vi "EPS-Remote Mode.vi"(8 "error in":errorcluster, 10 "Remote":bool, 11 "EPS Setting In":T1) -> (0 "error out":errorcluster, 3 "EPS Setting Out":T1)   [LabVIEW 2018]
uses:
  Data Def/EPS-Setting.ctl
  Data Def/EPS-Access Mode.ctl
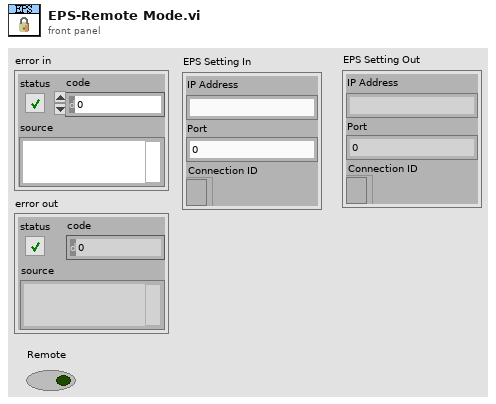
[diagram p1: front panel]
types:
  T1 = typedef "EPS-Setting.ctl" = cluster{"IP Address":string, "Port":u16, "Connection ID":refnum<k5>}
  T2 = typedef "EPS-Access Mode.ctl" = enum16{"Read", "Write"}
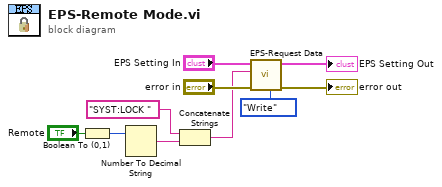
[diagram p0: block diagram]
diagram:
  n1 = Boolean To (0,1)(Boolean="Remote") -> (0, 1=w3:i16)
  n2 = Number To Decimal String(number=w3) -> (decimal integer string=w2:string)  [unwired: 1 in]
  n3 = Concatenate Strings("SYST:LOCK ", w2) -> (w1:string)
  n4 = call "EPS-Request Data.vi"("Access Mode"=EPS-Access_Mode."Write", "error in"="error in", "Requst Data"=w1, "EPS Setting In"="EPS Setting In") -> ("error out"=→"error out":errorcluster, "EPS Setting Out"=→"EPS Setting Out":T1)  [unwired: 5 in, 1 out]
